vi "IsMethodsCalled.vi"(8 "error in (no error)":errorcluster, 10 "ViRefnums":refnum<vi>[](array[refnum]), 11 "MockListImp in":refnum<class "ListImp_RefSpy.lvclass">) -> (0 "error out":errorcluster, 1 "Methods Called (OR)":bool, 2 "Methods Called (AND)":bool, 3 "MockListImp out":refnum<class "ListImp_RefSpy.lvclass">)   [LabVIEW 2009, in "ListImp_RefSpy.lvclass"]
uses:
  ListImp_RefSpy.lvclass
  RefnumGlobal.vi
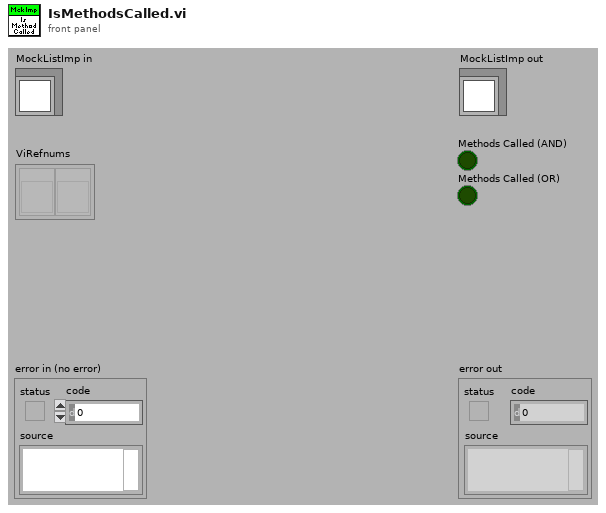
[diagram p1: front panel]
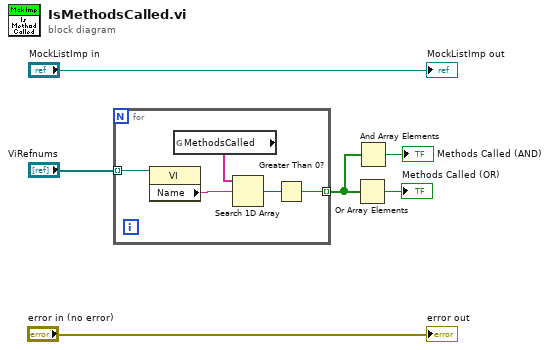
[diagram p0: block diagram]
diagram:
  n1 = for {
    tunnel: "ViRefnums" -> [w10] mode=indexing
    tunnel: [w7] -> w3 mode=indexing
    n2 = property class="VI"(reference=w10) -> ("Name"=w9:string)  [unwired: 1 in, 2 out]
    n3 = global read "RefnumGlobal.vi" "MethodsCalled"() -> (w11:string[])
    n4 = Search 1D Array(1D array=w11, element=w9) -> (index of element=w8:i32)  [unwired: 1 in]
    n5 = Greater Than 0?(x=w8) -> (x > 0?=w7:bool)
  }
  n6 = Or Array Elements(Boolean array=w3) -> (logical OR=→"Methods Called (OR)":bool)
  n7 = And Array Elements(Boolean array=w3) -> (logical AND=→"Methods Called (AND)":bool)
  "error out" <- "error in (no error)"
  "MockListImp out" <- "MockListImp in"
